vi "Check operation mode.vi"(7 "Quenched?":bool, 8 "Switch supercond [K]":dbl=4.0 format="%#_13g", 9 "Switch rezist [K]":dbl=5.0 format="%#_13g", 10 "Switch Heater":bool, 11 "Switch actual [K]":dbl) -> (3 "Magnet Mode":T1=enum."Switching")   [LabVIEW 2024, in "Magnet module.lvlib"]
doc: "Evaluates actual operation mode of magnet.\n\"Quenched\" is not implemented!"
uses:
  Magnet module.lvlib
  ctl/Magnet mode.ctl
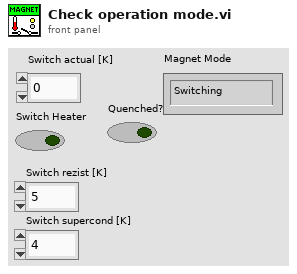
[diagram p1: front panel]
types:
  T1 = typedef "Magnet module.lvlib/Magnet mode.ctl" = enum16{"Persistant", "Switching", "Ramping", "Quenched"}
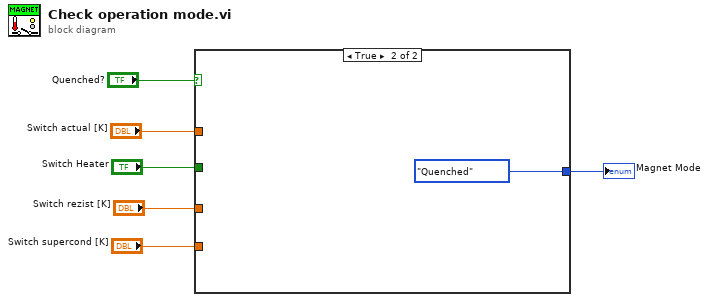
[diagram p0: block diagram]
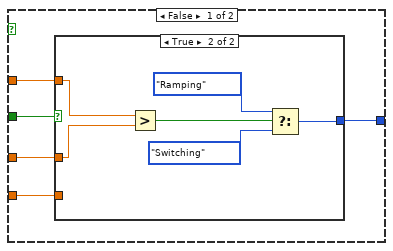
[diagram p2: hidden frame]
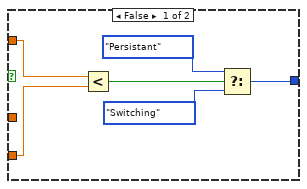
[diagram p3: hidden frame]
diagram:
  n1 = case shown="True" "Quenched?" {
    tunnel: [w11 Magnet_mode."Quenched" ("Mode 2")] -> w6
    tunnel: "Switch actual [K]" -> [w10 _]
    tunnel: "Switch Heater" -> [w9 _]
    tunnel: "Switch rezist [K]" -> [w8 _]
    tunnel: "Switch supercond [K]" -> [w7 _]
    frame False {
      n2 = case shown="True" w9 {
        tunnel: w10 -> [w17 w23]
        tunnel: [w15 w21] -> w11
        tunnel: w8 -> [_ w20]
        tunnel: w7 -> [w14 _]
        frame False {
          n3 = Less?(x=w17, y=w14) -> (x < y?=w16:bool)
          n4 = Select(t=Magnet_mode."Persistant" ("Mode 2"), s=w16, f=Magnet_mode."Switching" ("Mode 2")) -> (s? t:f=w15:T1)
        }
        frame True {
          n5 = Greater?(x=w23, y=w20) -> (0:w22:bool)
          n6 = Select(t=Magnet_mode."Ramping" ("Mode 2"), s=w22, f=Magnet_mode."Switching" ("Mode 2")) -> (s? t:f=w21:T1)
        }
      }
    }
    frame True {
    }
  }
  "Magnet Mode" <- w6
